vi "Populate Device Information Fields.vi"(3 "error in (no error)":errorcluster, 4 "Outputs":T1, 5 "Inputs":T2) -> (0 "error out":errorcluster)   [LabVIEW 2013, in "ACNET Monitor.lvlib"]
uses:
  ACNET Monitor.lvlib
  ACNET Devices.lvclass
  Find Device by Listbox Value.vi
  Find Range Check Result by Listbox Value.vi
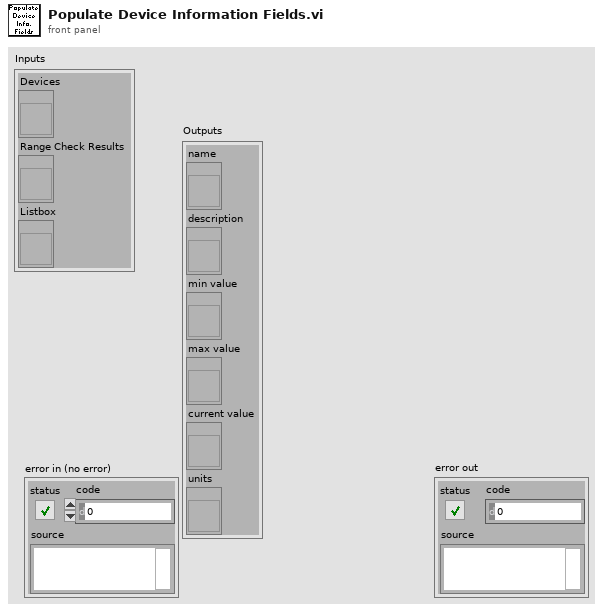
[diagram p1: front panel]
types:
  T1 = cluster{"name":refnum<vi>, "description":refnum<vi>, "min value":refnum<vi>, "max value":refnum<vi>, "current value":refnum<vi>, "units":refnum<vi>}
  T2 = cluster{"Devices":refnum<vi>, "Range Check Results":refnum<vi>, "Listbox":refnum<vi>}
  T3 = cluster{"name":string, "minValue":dbl, "maxValue":dbl, "units":string, "description":string, "ignoreMinValue":bool, "ignoreMaxValue":bool}
  T4 = cluster{"name":string, "value":dbl, "range state":i8}[]
  T5 = cluster{"name":string, "value":dbl, "range state":i8}
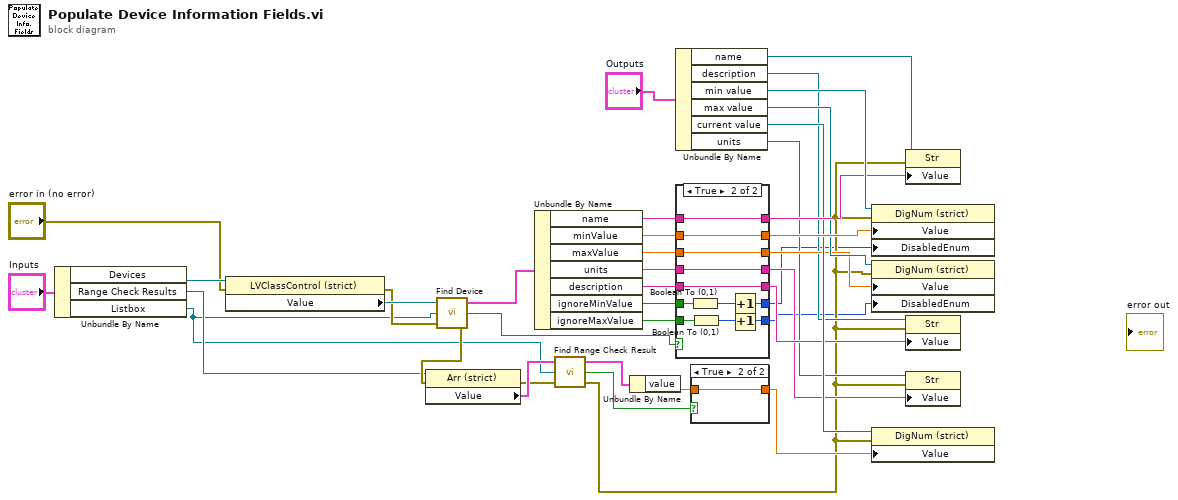
[diagram p0: block diagram]
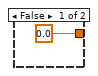
[diagram p2: hidden frame]
diagram:
  n1 = Unbundle By Name("Inputs") -> ("Devices"=w29:refnum<vi>, "Range Check Results"=w24:refnum<vi>, "Listbox"=w5:refnum<vi>)
  n2 = property class="LVClassControl (strict)"(reference=w29, error in="error in (no error)") -> (error out=w26:errorcluster, "Value"=w28:refnum<class "ACNET Devices.lvclass">)  [unwired: 1 out]
  n3 = call-poly "Find Device.vi"("error in (no error)"=w26, "Listbox"=w5, "ACNET Devices"=w28) -> ("error out"=w25:errorcluster, "Found?"=w34:bool, "ACNET Device Cluster"=w35:T3)
  n4 = property class="Arr (strict)"(reference=w24, error in=w25) -> (error out=w22:errorcluster, "Value"=w23:T4)  [unwired: 1 out]
  n5 = Unbundle By Name(w35) -> ("name"=w31:string, "minValue"=w38:dbl, "maxValue"=w37:dbl, "units"=w12:string, "description"=w10:string, "ignoreMinValue"=w4:bool, "ignoreMaxValue"=w3:bool)
  n6 = call-poly "Find Range Check Result.vi"("error in (no error)"=w22, "reference"=w5, "Range Check Results in"=w23) -> ("error out"=w6:errorcluster, "Found?"=w32:bool, "Range Check Result out"=w33:T5)
  n7 = Unbundle By Name(w33) -> ("value"=w36:dbl)
  n8 = Unbundle By Name("Outputs") -> ("name"=w13:refnum<vi>, "description"=w11:refnum<vi>, "min value"=w20:refnum<vi>, "max value"=w17:refnum<vi>, "current value"=w16:refnum<vi>, "units"=w8:refnum<vi>)
  n9 = case shown="True" w34 {
    tunnel: w38 -> [_ w49]
    tunnel: w37 -> [_ w48]
    tunnel: [_ w49] -> w18
    tunnel: [_ w48] -> w15
    tunnel: w31 -> [_ w47]
    tunnel: [_ w47] -> w19
    tunnel: [_ w46] -> w7
    tunnel: w12 -> [_ w46]
    tunnel: w10 -> [_ w45]
    tunnel: [_ w45] -> w9
    tunnel: w4 -> [_ w44]
    tunnel: w3 -> [_ w43]
    tunnel: [_ w40] -> w2
    tunnel: [_ w39] -> w1
    frame False {
    }
    frame True {
      n10 = Boolean To (0,1)(Boolean=w44) -> (0, 1=w42:i16)
      n11 = Boolean To (0,1)(Boolean=w43) -> (0, 1=w41:i16)
      n12 = Increment(x=w42) -> (x+1=w40:i16)
      n13 = Increment(x=w41) -> (x+1=w39:i16)
    }
  }
  n14 = case shown="True" w32 {
    tunnel: w36 -> [_ w51]
    tunnel: [0.0 ("minValue") w51] -> w14
    frame False {
    }
    frame True {
    }
  }
  n15 = property class="DigNum (strict)"(reference=w20, error in=w6, "Value"=w18, "DisabledEnum"=w2) -> ()  [unwired: 2 out]
  n16 = property class="DigNum (strict)"(reference=w17, error in=w6, "Value"=w15, "DisabledEnum"=w1) -> ()  [unwired: 2 out]
  n17 = property class="DigNum (strict)"(reference=w16, error in=w6, "Value"=w14) -> ()  [unwired: 2 out]
  n18 = property class="Str"(reference=w13, error in=w6, "Value"=w19) -> ()  [unwired: 2 out]
  n19 = property class="Str"(reference=w11, error in=w6, "Value"=w9) -> ()  [unwired: 2 out]
  n20 = property class="Str"(reference=w8, error in=w6, "Value"=w7) -> ()  [unwired: 2 out]
